vi "Get_KPRO_data_from_file.vi"(11 "Output File KPRO Test":path=path "c:/KPRO_001.txt") -> (0 "Last_height_of_box":dbl format="%.2f", 1 "Last_depth_to_water":dbl format="%.2f", 2 "Last_depth":dbl format="%.2f", 3 "Output_array":sgl[][](array[numeric]) format="%.2f")   [LabVIEW 2016]
uses:
  <vilib>/Utility/file.llb/Read Delimited Spreadsheet (DBL).vi
panel:
  out "report_header_length":i32
  out "Report_header_string":string
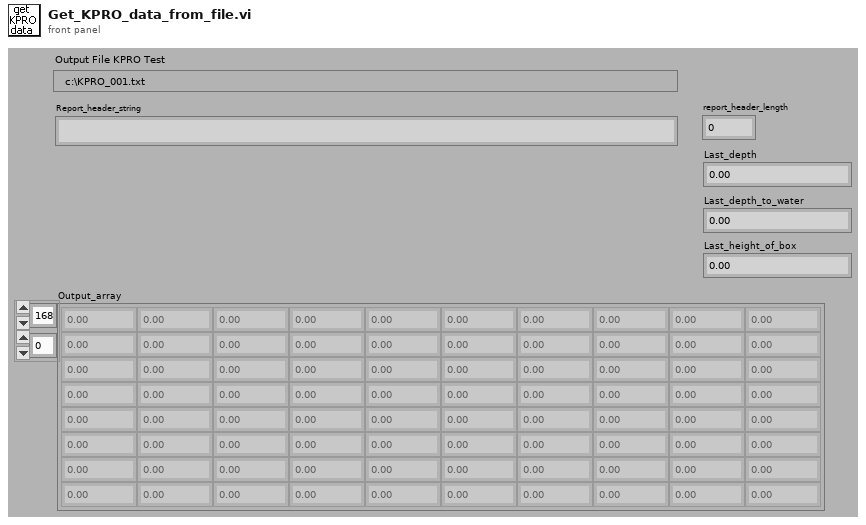
[diagram p1: front panel]
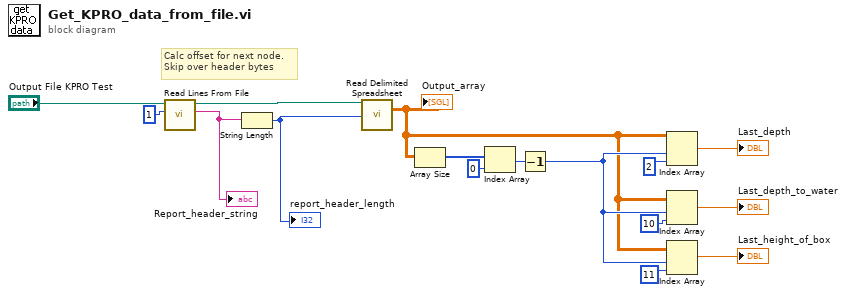
[diagram p0: block diagram]
diagram:
  # "Calc offset for next node.\nSkip over header bytes"
  n1 = call <vilib>:"Read Lines From File.vi"("file path (dialog if empty)"="Output File KPRO Test", "number of lines (all:-1)"=1) -> ("new file path (Not A Path if cancelled)"=w12:path, "line string"=w14:string)  [unwired: 4 in, 2 out]
  "Report_header_string" <- w14
  n2 = String Length(string=w14) -> (length=w16:i32)
  "report_header_length" <- w16
  n3 = call-poly <vilib>:"Read Delimited Spreadsheet.vi"("file path (dialog if empty)"=w12, "start of read offset (chars.:0)"=w16) -> ("all rows"=w3:dbl[][])  [unwired: 8 in, 5 out]
  "Output_array" <- w3
  n4 = Array Size(array=w3) -> (size(s)=w10:i32[])
  n5 = Index Array(array=w10, index=0) -> (element=w8:i32)
  n6 = Decrement(x=w8) -> (x-1=w6:i32)
  n7 = Index Array(array=w3, index (row)=w6, index (col)=2 ("index")) -> (element=→"Last_depth":dbl)
  n8 = Index Array(array=w3, index (row)=w6, index (col)=10 ("disabled index (col)")) -> (element=→"Last_depth_to_water":dbl)
  n9 = Index Array(array=w3, index (row)=w6, index (col)=11 ("index")) -> (element=→"Last_height_of_box":dbl)
